vi "VariantToRefnum.vi"(8 "error in (no error)":errorcluster, 11 "Refnum":variant) -> (0 "error out":errorcluster, 1 "strict type":variant, 2 "type":string, 3 "value":string)   [LabVIEW 2019, in "BlueVariantView.lvlib"]
uses:
  BlueVariantView.lvlib
  <vilib>/Utility/Data Type/NI_Data Type.lvlib
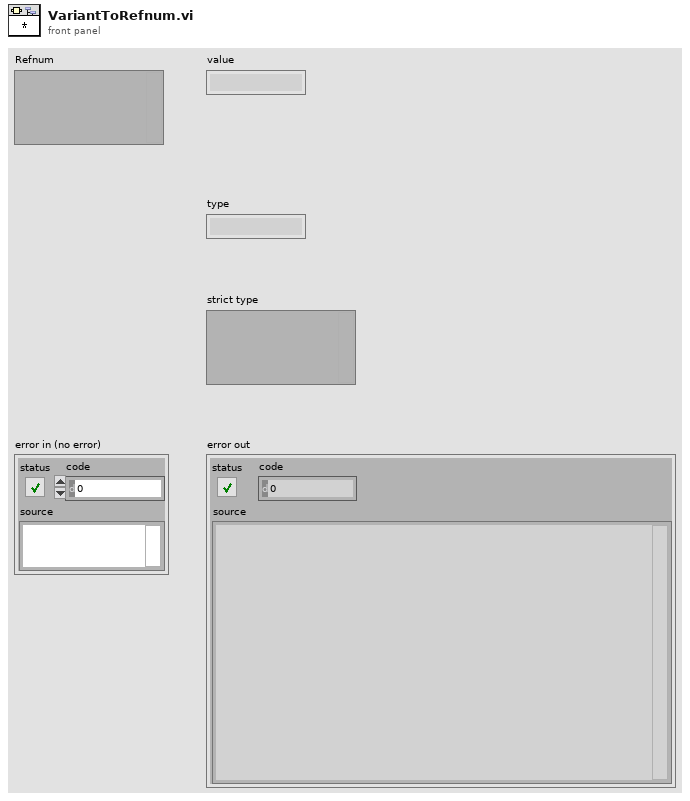
[diagram p1: front panel]
types:
  T1 = typedef "NI_Data Type.lvlib/Refnum Type.ctl" = enum16{"NotARefnum", "UnknownRefnum", "Generic", "Datalog", "ByteStream", "Device", "Occurence", "TCPNetConnection", "Auto", "Menu", "Imaq", "Hardware", "DataSocket", "Visa", "IVI", "UDPNetConnection", "Notifier", "Queue", "Irda", "EventReg", "DotNet", "UserEvent", "Callback", "UNUSED_EMPTY_POSITION", "BlueToothNetConnection", "LVObjApp", "LVObjVI", "LVObjUnknown", "GenericClass", "UserDefinedRefnumTag", "DataValue", "RT FIFO", "TDMS File", "PythonSessionRefnum"}
  T2 = enum32{"invalid VI type", "Standard VI", "Control VI", "Global VI", "Polymorphic VI", "Configuration VI", "SubSystem", "Facade VI", "Method VI", "Statechart Diagram VI"}
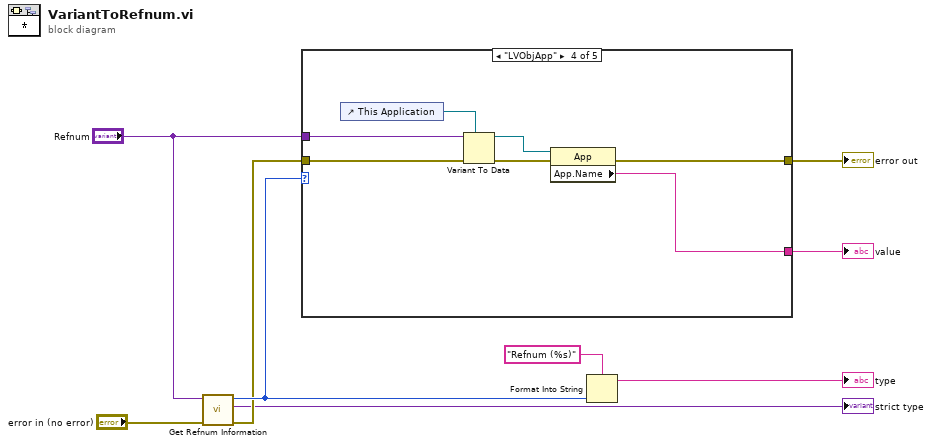
[diagram p0: block diagram]
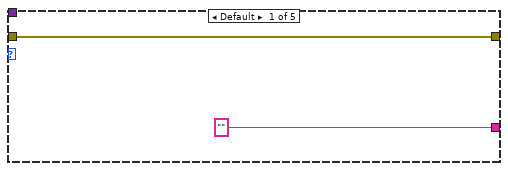
[diagram p2: hidden frame]
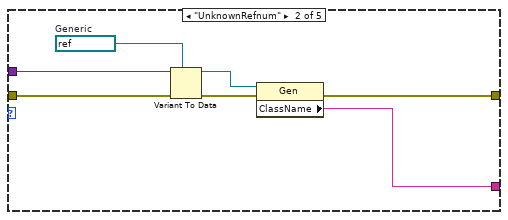
[diagram p3: hidden frame]
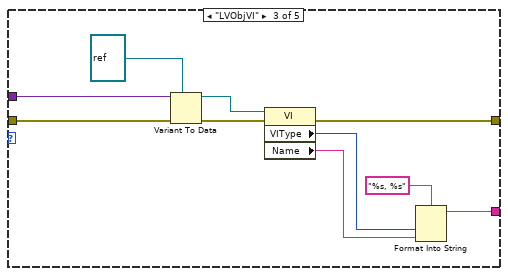
[diagram p4: hidden frame]
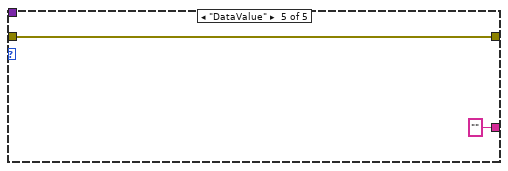
[diagram p5: hidden frame]
diagram:
  n1 = call <vilib>:"Get Refnum Information.vi"("error in (no error)"="error in (no error)", "variant"="Refnum") -> ("error out"=w3:errorcluster, "strict type"=→"strict type":variant, "reference type"=w7:T1)  [unwired: 6 in, 1 out]
  n2 = case shown="\"LVObjApp\"" w7 {
    tunnel: "Refnum" -> [_ w17 w27 w34 _]
    tunnel: ["" ("ClassName") w15 w19 w29 "" ("App.Name")] -> w4
    tunnel: w3 -> [w11 w14 w26 w33 w37]
    tunnel: [w11 w12 w24 w31 w37] -> w1
    frame Default {
    }
    frame "UnknownRefnum" {
      w16 = refnum<vi> refnum  # Generic
      n3 = Variant To Data(error in=w14, type=w16, Variant=w17) -> (data=w18:refnum<vi>, error out=w13:errorcluster)
      n4 = property class="Gen"(reference=w18, error in=w13) -> (error out=w12:errorcluster, "ClassName"=w15:string)  [unwired: 1 out]
    }
    frame "LVObjVI" {
      n5 = Variant To Data(error in=w26, type=refnum<vi> refnum ("vi reference"), Variant=w27) -> (data=w28:refnum<vi>, error out=w25:errorcluster)
      n6 = property class="VI"(reference=w28, error in=w25) -> (error out=w24:errorcluster, "VIType"=w21:T2, "Name"=w20:string)  [unwired: 1 out]
      n7 = Format Into String(format string="%s, %s", w21, w20) -> (resulting string=w19:string)  [unwired: 2 in, 1 out]
    }
    frame "LVObjApp" {
      n8 = control-ref of="This Application"() -> (w30:refnum<vi>)
      n9 = Variant To Data(error in=w33, type=w30, Variant=w34) -> (data=w35:refnum<vi>, error out=w32:errorcluster)
      n10 = property class="App"(reference=w35, error in=w32) -> (error out=w31:errorcluster, "App.Name"=w29:string)  [unwired: 1 out]
    }
    frame "DataValue" {
    }
  }
  "error out" <- w1
  "value" <- w4
  n11 = Format Into String(format string="Refnum (%s)", w7) -> (resulting string=→"type":string)  [unwired: 2 in, 1 out]
